vi "传感器数据.vi"() -> (3 "传感器读数":T1 {"电缸压力" format="%#.3f"; "输出扭矩(大)" format="%#.3f"; "输出扭矩(小)" format="%#.3f"; "输入扭矩" format="%#.3f"; "电缸位移" format="%#.3f"; "工装移载位移" format="%#.3f"; "输入移载位移" format="%#.3f"; "输入旋转位移" format="%#.3f"})   [LabVIEW 2020]
uses:
  Libraries/S7/S7.lvlib
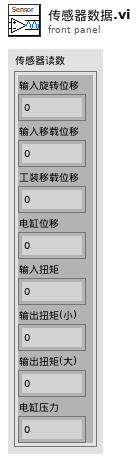
[diagram p1: front panel]
types:
  T1 = cluster{"输入旋转位移":sgl, "输入移载位移":sgl, "工装移载位移":sgl, "电缸位移":sgl, "输入扭矩":sgl, "输出扭矩(小)":sgl, "输出扭矩(大)":sgl, "电缸压力":sgl}
  T2 = cluster{"输入轴扭矩":dbl, "输出轴扭矩小量程":dbl, "输出轴扭矩大量程":dbl}
  T3 = typedef "S7.lvlib/Read_Data (Reply Payload)--cluster.ctl" = cluster{"读取成功":bool, "数据":u32[], "Read_Data_error":errorcluster}
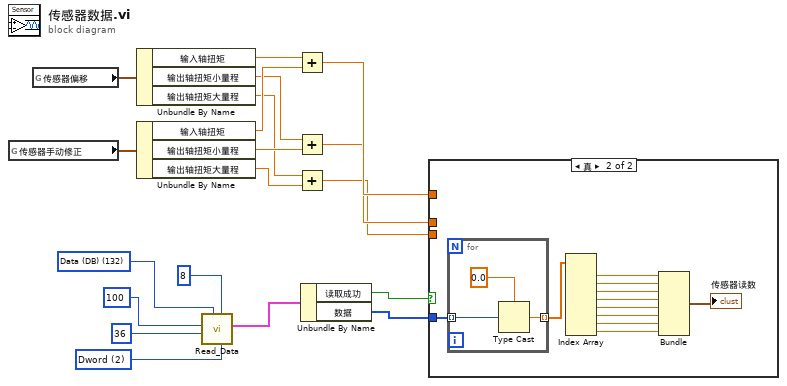
[diagram p0: block diagram]
diagram:
  w16 = u16 2 items=["byte", "word", "Dword"] ("数据类型")
  w17 = u8 132 items=["I/O (P)"=128, "Input (I)"=129, "Output (Q)"=130, "Bit Memory (M)"=131, "Data (DB)"=132, "Instance Data (DI)"=133, "Local Data (L)"=134, "Predecessor Local Data (VL)"=135] ("寄存器类型")
  n1 = global read "传感器偏移.vi" "传感器手动修正"() -> (w10:T2)
  n2 = global read "传感器偏移.vi" "传感器偏移"() -> (w11:T2)
  n3 = Unbundle By Name(w11) -> ("输入轴扭矩"=w9:dbl, "输出轴扭矩小量程"=w7:dbl, "输出轴扭矩大量程"=w5:dbl)
  n4 = Unbundle By Name(w10) -> ("输入轴扭矩"=w8:dbl, "输出轴扭矩小量程"=w6:dbl, "输出轴扭矩大量程"=w4:dbl)
  n5 = call "Read_Data.vi"("数据类型"=w16, "读取长度"=u16 8, "寄存器类型"=w17, "起始地址"=u32 36, "DB #"=u16 100) -> ("Reply Payload"=w14:T3)  [unwired: 4 in, 2 out]
  n6 = Add(x=w9, y=w8) -> (x+y=w3:dbl)
  n7 = Add(x=w7, y=w6) -> (x+y=w2:dbl)
  n8 = Add(x=w5, y=w4) -> (x+y=w1:dbl)
  n9 = Unbundle By Name(w14) -> ("读取成功"=w12:bool, "数据"=w13:u32[])
  n10 = case shown="真" w12 {
    tunnel: w13 -> [_ w30]
    tunnel: w3 -> [_ _]
    tunnel: w2 -> [_ _]
    tunnel: w1 -> [_ _]
    frame False {
    }
    frame True {
      n11 = for {
        tunnel: w30 -> [w32] mode=indexing
        tunnel: [w31] -> w29 mode=indexing
        n12 = Type Cast(type=sgl 0.0, x=w32) -> (*(type *) &x=w31:sgl)
      }
      n13 = Index Array(array=w29) -> (element #1=w28:sgl, element #2=w27:sgl, element #3=w26:sgl, element #4=w25:sgl, element #5=w23:sgl, element #6=w22:sgl, element #7=w21:sgl, element #8=w24:sgl)  [unwired: 8 in]
      n14 = Bundle(w28, w27, w26, w25, w23, w22, w21, w24) -> (→"传感器读数":cluster{sgl, sgl, sgl, sgl, sgl, sgl, sgl, sgl})  [unwired: 1 in]
    }
  }
